vi "9.4.обработка файла натекания.vi"() -> (0 "all rows":string[][](array[string]), 1 "output cluster":T1, 3 "array_graph out":cluster{"String":dbl, "String":dbl}[](array[cluster]), 5 "path_naton":path)   [LabVIEW 2016, in "Library.lvlib"]
uses:
  <vilib>/Utility/file.llb/Read From Spreadsheet File (string).vi
  Granule-2000AT/PC/Library.lvlib
panel:
  in  "Величина течи\n(torr*mkL/sec)":string caption="Вакуум в камере\nPT2 (torr)"
  in  "Время проверки (sec)":string caption="Вакуум в камере\nPT2 (torr)"
  in  "Завершение проверки":string caption="Вакуум в камере\nPT2 (torr)"
  in  "Начало проверки":string caption="Вакуум в камере\nPT2 (torr)"
  in  "array_graph":cluster{"String":dbl, "String":dbl}[](array[cluster])
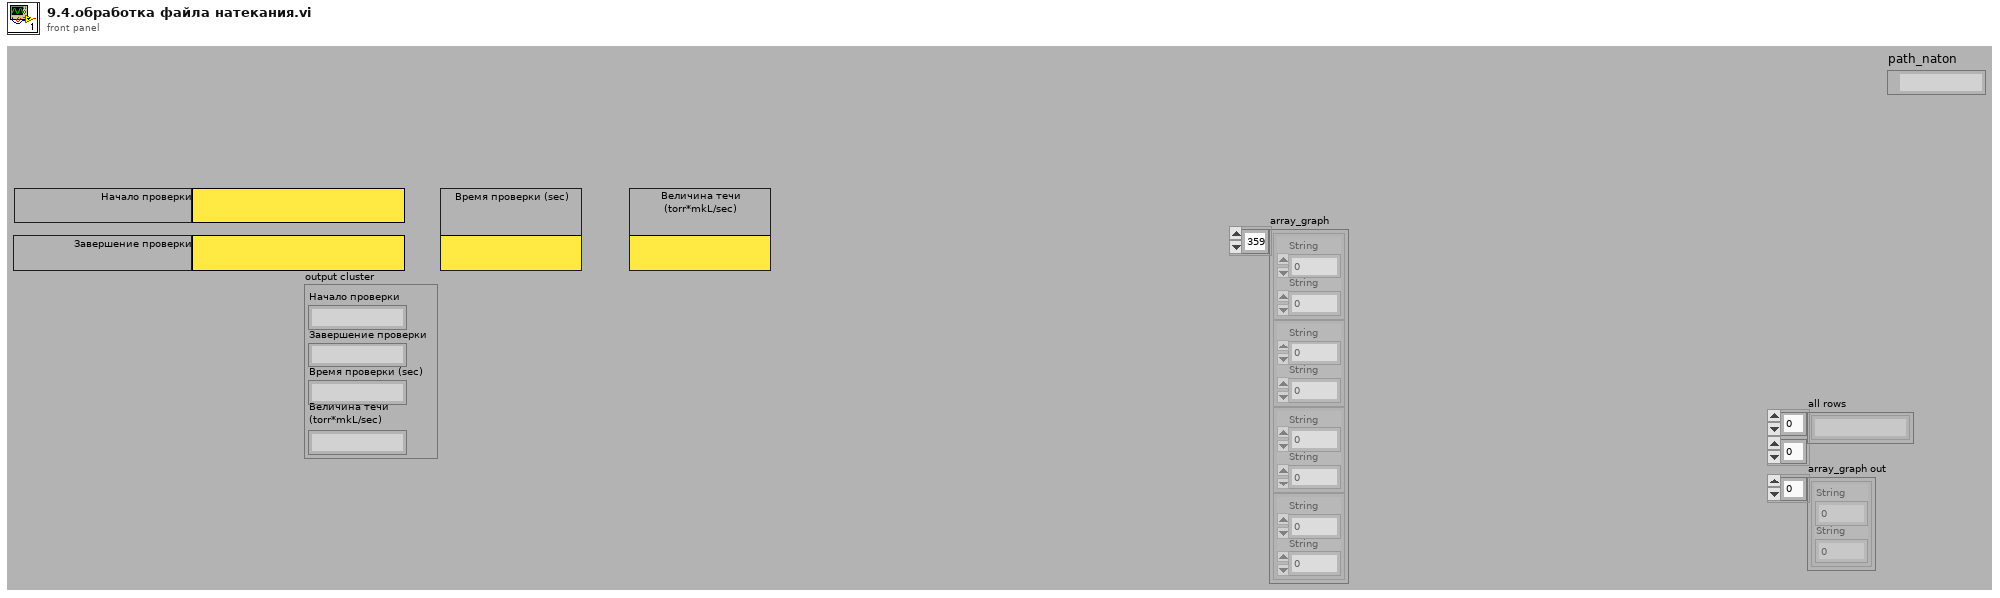
[diagram p1: front panel]
types:
  T1 = cluster{"Начало проверки":string, "Завершение проверки":string, "Время проверки (sec)":string, "Величина течи\n(torr*mkL/sec)":string}
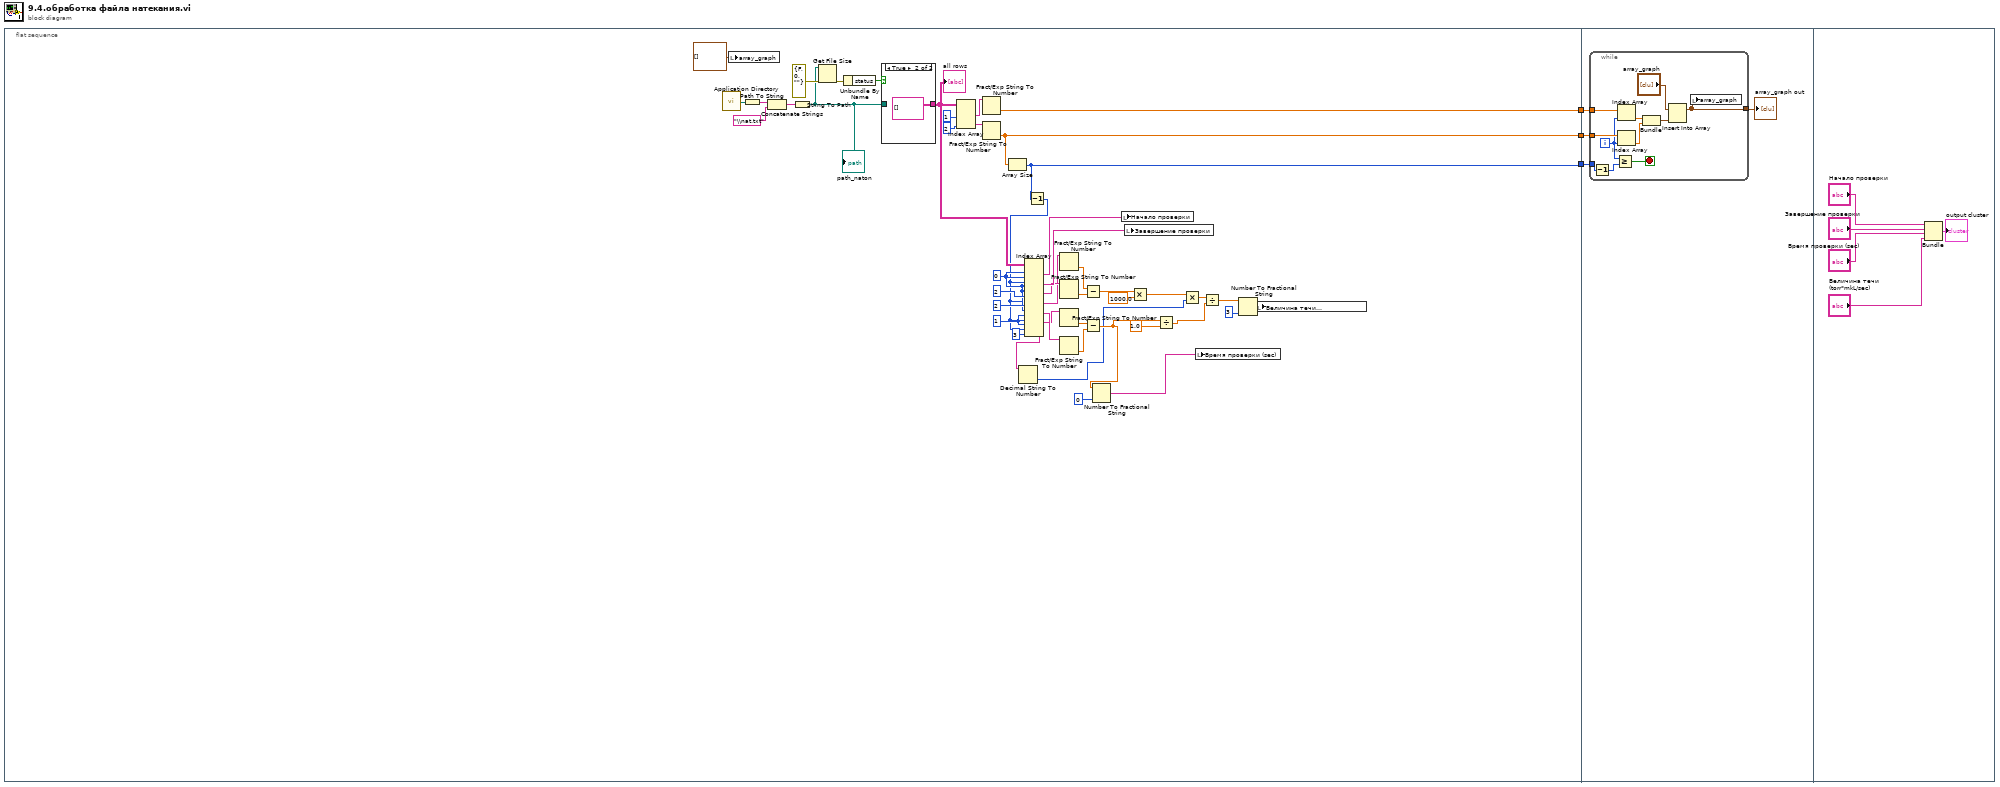
[diagram p0: block diagram]
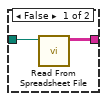
[diagram p2: hidden frame]
diagram:
  n1 = flat-sequence {
    tunnel: [w38] -> w3
    tunnel: [w37] -> w2
    tunnel: [w13] -> w1
    tunnel: w3 -> [w57]
    tunnel: w2 -> [w56]
    tunnel: w1 -> [w55]
    frame #0 {
      w24 = 1 ("disabled index (col)")
      w25 = 0 ("index (row)")
      n2 = call <vilib>:"Application Directory.vi"() -> ("Application Directory"=w50:path)
      n3 = local write "array_graph"(cluster{"String":dbl, "String":dbl}[] [] ("array")) -> ()
      n4 = Path To String(path=w50) -> (string=w49:string)
      n5 = Concatenate Strings(w49, "\\nat.txt" ("string")) -> (w47:string)
      n6 = String To Path(string=w47) -> (path=w43:path)
      "path_naton" <- w43
      n7 = Get File Size(file=w43, error in=errorcluster {"status"=FALSE, "code"=0, "source"=""}) -> (0:w45:errorcluster)  [unwired: 2 out]
      n8 = Unbundle By Name(w45) -> ("status"=w44:bool)
      n9 = case shown="True" w44 {
        tunnel: w43 -> [w52 _]
        tunnel: [w51 string[][] [] ("all rows")] -> w14
        frame False {
          n10 = call-poly <vilib>:"Read From Spreadsheet File.vi"("file path (dialog if empty)"=w52) -> ("all rows"=w51:string[][])  [unwired: 6 in, 4 out]
        }
        frame True {
        }
      }
      "all rows" <- w14
      n11 = Index Array(array=w14, index (col) #1=1 ("disabled index (col)"), index (col) #2=2 ("index (col)")) -> (element #1=w40:string[], element #2=w39:string[])  [unwired: 2 in]
      n12 = Fract/Exp String To Number(string=w40) -> (number=w38:dbl[])  [unwired: 3 in, 1 out]
      n13 = Fract/Exp String To Number(string=w39) -> (number=w37:dbl[])  [unwired: 3 in, 1 out]
      n14 = Array Size(array=w37) -> (size(s)=w13:i32)
      n15 = Decrement(x=w13) -> (x-1=w7:i32)
      n16 = Index Array(array=w14, index (row) #1=w25, index (col) #1=w25, index (row) #2=w7, index (col) #2=w25, index (row) #3=w25, index (col) #3=2 ("disabled index (col)"), index (row) #4=w7, index (col) #4=2 ("index (col)"), index (row) #5=w25, index (col) #5=w24, index (row) #6=w7, index (col) #6=w24, index (row) #7=w7, index (col) #7=3 ("disabled index (col)")) -> (element #1=w35:string, element #2=w34:string, element #3=w32:string, element #4=w30:string, element #5=w23:string, element #6=w22:string, element #7=w5:string)
      n17 = Decimal String To Number(string=w5) -> (number=w4:i32)  [unwired: 2 in, 1 out]
      n18 = Fract/Exp String To Number(string=w30) -> (number=w29:dbl)  [unwired: 3 in, 1 out]
      n19 = Fract/Exp String To Number(string=w32) -> (number=w28:dbl)  [unwired: 3 in, 1 out]
      n20 = Fract/Exp String To Number(string=w22) -> (number=w21:dbl)  [unwired: 3 in, 1 out]
      n21 = Fract/Exp String To Number(string=w23) -> (number=w20:dbl)  [unwired: 3 in, 1 out]
      n22 = Subtract(x=w29, y=w28) -> (x-y=w27:dbl)
      n23 = Subtract(x=w21, y=w20) -> (x-y=w10:dbl)
      n24 = Number To Fractional String(number=w10, precision (6)=i16 0) -> (F-format string=w11:string)  [unwired: 2 in]
      n25 = local write "Начало проверки"(w35) -> ()
      n26 = local write "Завершение проверки"(w34) -> ()
      n27 = Multiply(x=w27, y=1000.0) -> (x*y=w19:dbl)
      n28 = Divide(x=w10, y=1.0) -> (x/y=w8:dbl)
      n29 = Multiply(x=w19, y=w4) -> (x*y=w18:dbl)
      n30 = local write "Время проверки (sec)"(w11) -> ()
      n31 = Divide(x=w18, y=w8) -> (x/y=w17:dbl)
      n32 = Number To Fractional String(number=w17, precision (6)=i16 3) -> (F-format string=w15:string)  [unwired: 2 in]
      n33 = local write "Величина течи\n(torr*mkL/sec)"(w15) -> ()
    }
    frame #1 {
      n34 = while {
        tunnel: w57 -> [w68]
        tunnel: w56 -> [w67]
        tunnel: w55 -> [w58]
        tunnel: [w60] -> w54
        i -> [w62]
        stop <- w61 stop-if-true
        n35 = Decrement(x=w58) -> (x-1=w59:i32)
        n36 = Greater Or Equal?(x=w62, y=w59) -> (x >= y?=w61:bool)
        n37 = Index Array(array=w68, index=w62) -> (element=w66:dbl)
        n38 = Index Array(array=w67, index=w62) -> (element=w65:dbl)
        n39 = Bundle("String"=w66, "String"=w65) -> (w64:cluster{"String":dbl, "String":dbl})  [unwired: 1 in]
        n40 = Insert Into Array(array="array_graph", new element=w64) -> (w60:cluster{"String":dbl, "String":dbl}[])  [unwired: 1 in]
        n41 = local write "array_graph"(w60) -> ()
      }
      "array_graph out" <- w54
    }
    frame #2 {
      n42 = Bundle("Начало проверки"="Начало проверки", "Завершение проверки"="Завершение проверки", "Время проверки (sec)"="Время проверки (sec)", "Величина течи\n(torr*mkL/sec)"="Величина течи\n(torr*mkL/sec)") -> (→"output cluster":T1)  [unwired: 1 in]
    }
  }
